vi "Identify.vi"(8 "error in (no error)":errorcluster, 11 "NULL_ADAPTER in":refnum<class "Null Adapter.lvclass">) -> (0 "error out":errorcluster, 2 "Plugin is Valid":bool, 3 "NULL_ADAPTER out":refnum<class "Null Adapter.lvclass">)   [LabVIEW 2018, in "Null Adapter.lvlib" / "Null Adapter.lvclass"]
uses:
  Null Adapter.lvclass
  c:/Sequence Automation/Plugins/Measurement Interface.lvlibp/Measurement Interface.lvclass
  Plugins/Measurement Interface.lvlibp/Private Methods/Measurement Definition Entry/Read Measurement Definition Entry.vi
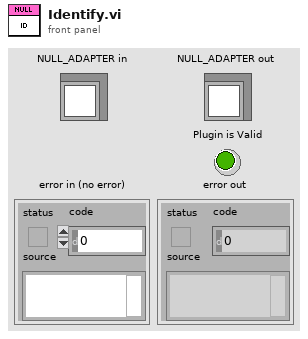
[diagram p1: front panel]
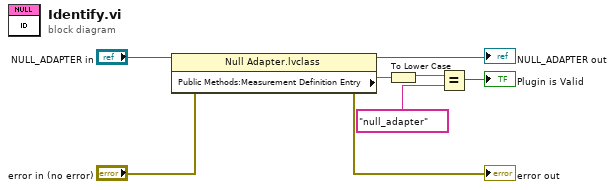
[diagram p0: block diagram]
diagram:
  n1 = property class="Null Adapter.lvclass"(reference="NULL_ADAPTER in", error in="error in (no error)") -> (reference out=→"NULL_ADAPTER out":refnum<class "Null Adapter.lvclass">, error out=→"error out":errorcluster, "Public Methods:Measurement Definition Entry"=w7:string)
  n2 = To Lower Case(string=w7) -> (all lower case string=w5:string)
  n3 = Equal?(x=w5, y="null_adapter") -> (x = y?=→"Plugin is Valid":bool)
